vi "UTIL_CalcCalCoef.vi"(8 "LKe":dbl, 9 "SHi":dbl, 10 "MLo":dbl, 11 "MHi":dbl) -> (2 "B":dbl, 3 "M":dbl)   [LabVIEW 2024]
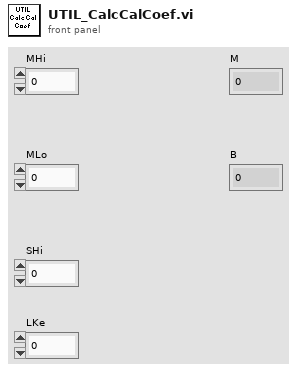
[diagram p1: front panel]
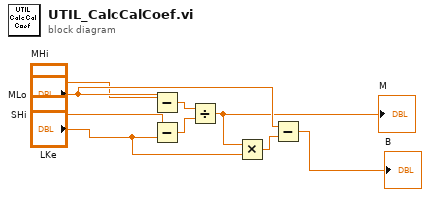
[diagram p0: block diagram]
diagram:
  n1 = Subtract(x="MHi", y="MLo") -> (x-y=w1:dbl)
  n2 = Subtract(x="SHi", y="LKe") -> (x-y=w2:dbl)
  n3 = Divide(x=w1, y=w2) -> (x/y=w5:dbl)
  "M" <- w5
  n4 = Multiply(x=w5, y="LKe") -> (x*y=w3:dbl)
  n5 = Subtract(x="MLo", y=w3) -> (x-y=→"B":dbl)
